vi "time s to us.vi"(10 "time (s)":dbl) -> (2 "time (us)":fxp<+,48,48>)   [LabVIEW 2017]
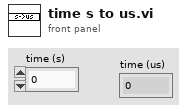
[diagram p1: front panel]
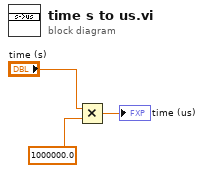
[diagram p0: block diagram]
diagram:
  n1 = Multiply(x="time (s)", y=1000000.0) -> (x*y=→"time (us)":dbl)
